vi "Get Items Data.vi"(7 "Calling VI Ref":refnum<vi>, 8 "error in (no error)":errorcluster, 11 "Items":refnum<class "Item.lvclass">[](array[class])) -> (0 "error out":errorcluster, 2 "Cancelled?":bool, 3 "Items out":refnum<class "Item.lvclass">[](array[class]))   [LabVIEW 2020, in "VI Properties Editor.lvlib"]
doc: "Gets property data for <B>Items</B>."
uses:
  VI Properties Editor.lvlib
  Classes/Item/Item.lvclass
  Classes/Loading Dialog/Loading Dialog.lvclass
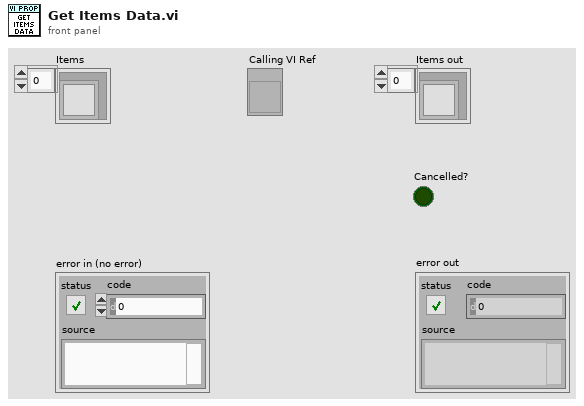
[diagram p1: front panel]
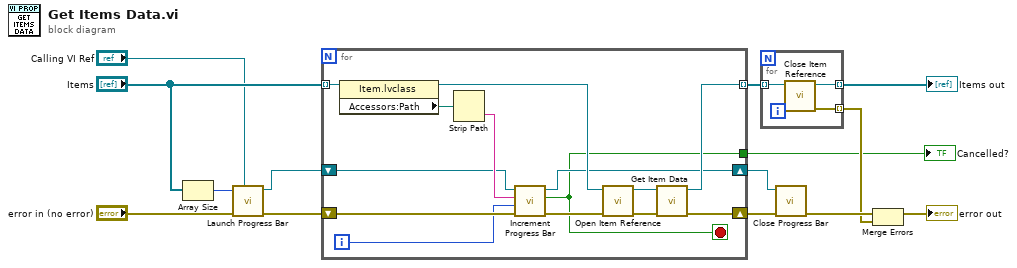
[diagram p0: block diagram]
diagram:
  n1 = Array Size(array="Items") -> (size(s)=w5:i32)
  n2 = call "Launch Progress Bar.vi"("Calling VI Ref"="Calling VI Ref", "error in (no error)"="error in (no error)", "Total Count"=w5) -> ("error out"=w11:errorcluster, "Progress Bar Dialog"=w4:refnum<class "Loading Dialog.lvclass">)  [unwired: 7 in]
  n3 = for {
    tunnel: "Items" -> [w22] mode=indexing
    shift-right: [w24] -> w14
    shift-left: w11 -> [w26]
    tunnel: [w23] -> w9 mode=indexing
    shift-right: [w20] -> w3
    shift-left: w4 -> [w15]
    tunnel: [w16] -> w1
    i -> [w17]
    stop <- w16 stop-if-true
    n4 = property class="Item.lvclass"(reference=w22) -> (reference out=w28:refnum<class "Item.lvclass">, "Accessors:Path"=w19:path)  [unwired: 1 in, 1 out]
    n5 = Strip Path(path=w19) -> (name=w18:string)  [unwired: 1 out]
    n6 = call "Increment Progress Bar.vi"("error in (no error)"=w26, "Step Number (0: inc)"=w17, "Step Name (\"\")"=w18, "Progress Bar Dialog in"=w15) -> ("error out"=w25:errorcluster, "Cancelled?"=w16:bool, "Progress Bar Dialog out"=w20:refnum<class "Loading Dialog.lvclass">)  [unwired: 5 in]
    n7 = call-dynamic "Open Item Reference.vi"("error in (no error)"=w25, "Item in"=w28) -> ("error out"=w27:errorcluster, "Item out"=w21:refnum<class "Item.lvclass">)  [unwired: 8 in]
    n8 = call-dynamic "Get Item Data.vi"("error in (no error)"=w27, "Item in"=w21) -> ("error out"=w24:errorcluster, "Item out"=w23:refnum<class "Item.lvclass">)  [unwired: 8 in]
  }
  "Cancelled?" <- w1
  n9 = for {
    tunnel: w9 -> [w30] mode=indexing
    tunnel: [w29] -> w8 mode=indexing
    tunnel: [w31] -> w7 mode=indexing
    n10 = call-dynamic "Close Item Reference.vi"("Item in"=w30) -> ("error out"=w31:errorcluster, "Item out"=w29:refnum<class "Item.lvclass">)  [unwired: 9 in]
  }
  "Items out" <- w8
  n11 = call "Close Progress Bar.vi"("error in (no error)"=w14, "Progress Bar Dialog"=w3) -> ("error out"=w10:errorcluster)  [unwired: 9 in]
  n12 = Merge Errors(w10, w7) -> (→"error out":errorcluster)
